vi "Measure_DUT_Capacitance.vi"(8 "error in":errorcluster, 9 "SoakTime":u16, 10 "AutoSoakFlag":u16) -> (0 "error out":errorcluster, 1 "data":string, 2 "Capacitance Data (in pF)":dbl format="%#.8g", 3 "Measure$":string)   [LabVIEW 2020]
uses:
  <vilib>/express/express arith-compare/Formula/XNode/ExpressFormulaBlockNode.xnode
panel:
  out "Total Time":i32
  out "Count":i32
  out "Qual 2 Data":dbl
  out "Qual Data":dbl
  out "Max Count":u32
  in  "DeltaCap!":dbl
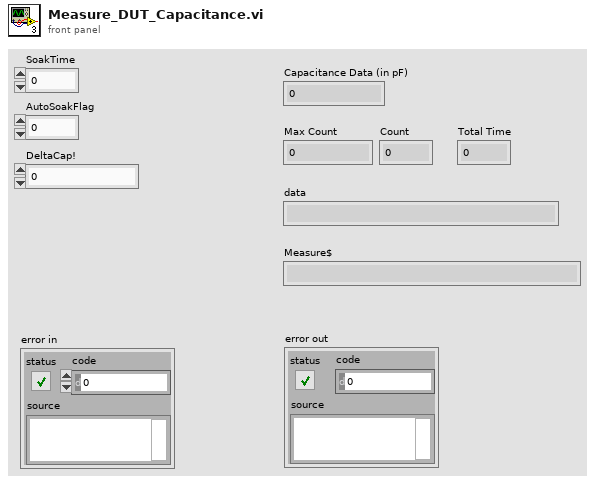
[diagram p1: front panel]
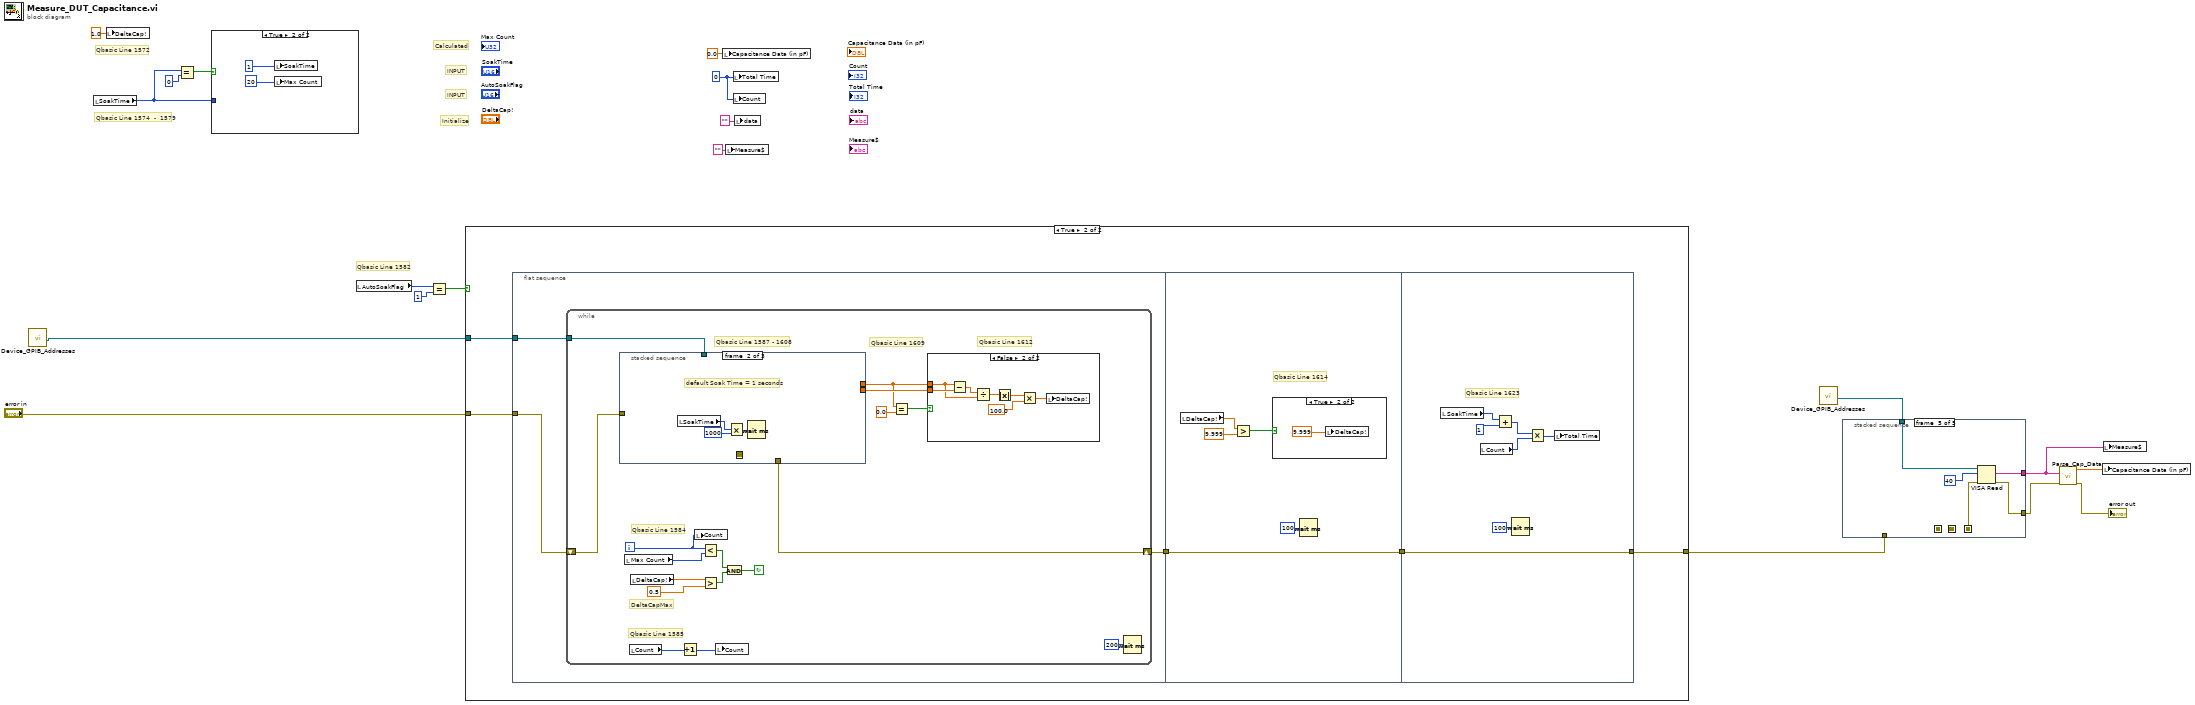
[diagram p0: block diagram]
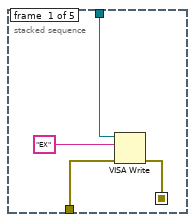
[diagram p2: hidden frame]
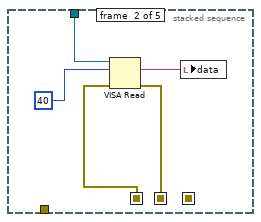
[diagram p3: hidden frame]
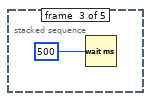
[diagram p4: hidden frame]
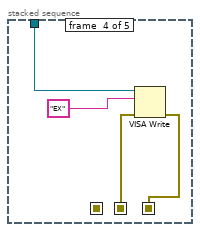
[diagram p5: hidden frame]
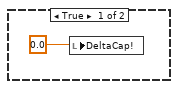
[diagram p7: hidden frame]
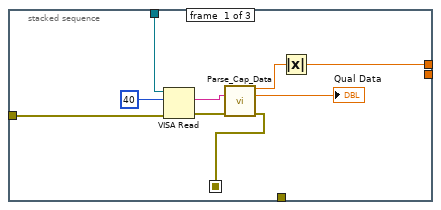
[diagram p8: hidden frame]
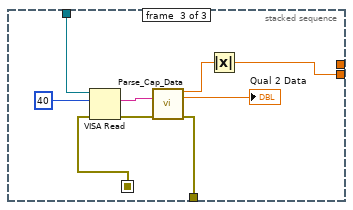
[diagram p9: hidden frame]
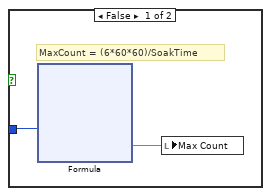
[diagram p11: hidden frame]
diagram:
  w4 = 0 ("Total Time")
  # "Initialize"
  # "Qbasic Line 1582"
  # "Calculated"
  # "Qbasic Line 1574  -  1579"
  # "INPUT"
  # "INPUT"
  # "Qbasic Line 1572"
  n1 = call "Device_GPIB_Addresses.vi"() -> ("HP 4275A Address"=w13:refnum<visa-resource-name>)  [unwired: 9 in, 2 out]
  n2 = local read "SoakTime"() -> (w8:u16)
  n3 = local write "DeltaCap!"(1.0 ("DeltaCap!")) -> ()
  n4 = Equal?(x=w8, y=0) -> (x = y?=w19:bool)
  n5 = case shown="True" w19 {
    tunnel: w8 -> [w21 _]
    frame False {
      # "MaxCount = (6*60*60)/SoakTime"
      n6 = xnode "Formula"("X1"=w21) -> ("Result"=w20:dbl)  [unwired: 1 in, 1 out]
      n7 = local write "Max Count"(w20) -> ()
    }
    frame True {
      n8 = local write "SoakTime"(1) -> ()
      n9 = local write "Max Count"(20) -> ()
    }
  }
  n10 = local read "AutoSoakFlag"() -> (w9:u16)
  n11 = Equal?(x=w9, y=u16 1) -> (x = y?=w16:bool)
  n12 = case shown="True" w16 {
    tunnel: "error in" -> [w32 w37]
    tunnel: [w32 w36] -> w15
    tunnel: w13 -> [_ w35]
    frame False {
    }
    frame True {
      n13 = flat-sequence {
        tunnel: w37 -> [w40]
        tunnel: w35 -> [w38]
        tunnel: [w39] -> w34
        tunnel: w34 -> [w91]
        tunnel: [w91] -> w33
        tunnel: [w99] -> w36
        tunnel: w33 -> [w99]
        frame #0 {
          n14 = while {
            tunnel: w38 -> [w46]
            shift-right: [w54] -> w39
            shift-left: w40 -> [w55]
            i -> [w41]
            stop <- w56 continue-if-true
            # "Qbasic Line 1609"
            # "Qbasic Line 1587 - 1608"
            # "Qbasic Line 1612"
            # "Qbasic Line 1585"
            # "Qbasic Line 1584"
            # "DeltaCapMax"
            n15 = stacked-sequence {
              seq-local: [w72 _ _] -> [_ _ w79]
              tunnel: w55 -> [w68 _ _]
              tunnel: [_ _ w85] -> w54
              tunnel: [_ _ w83] -> w53
              tunnel: [w71 _ _] -> w52
              tunnel: w46 -> [w70 _ w82]
              frame #0 {
                n16 = VISA Read(VISA resource name=w70, byte count=40, error in (no error)=w68) -> (read buffer=w67:string, error out=w66:errorcluster)  [unwired: 2 out]
                n17 = call "Parse_Cap_Data.vi"("Measure$"=w67, "error in"=w66) -> ("Capacitance Data (in pF)"=w74:dbl, "Qual Data"=→"Qual Data":dbl, "error out"=w72:errorcluster)  [unwired: 8 in, 3 out]
                n18 = Absolute Value(x=w74) -> (abs(x)=w71:dbl)
              }
              frame #1 {
                # "default Soak Time = 1 seconds"
                n19 = local read "SoakTime"() -> (w77:u16)
                n20 = Multiply(x=w77, y=u16 1000) -> (x*y=w75:u16)
                n21 = Wait (ms)(milliseconds to wait=w75) -> ()  [unwired: 1 out]
              }
              frame #2 {
                n22 = VISA Read(VISA resource name=w82, byte count=40, error in (no error)=w79) -> (read buffer=w78:string, error out=w80:errorcluster)  [unwired: 2 out]
                n23 = call "Parse_Cap_Data.vi"("Measure$"=w78, "error in"=w80) -> ("Capacitance Data (in pF)"=w86:dbl, "Qual Data"=→"Qual 2 Data":dbl, "error out"=w85:errorcluster)  [unwired: 8 in, 3 out]
                n24 = Absolute Value(x=w86) -> (abs(x)=w83:dbl)
              }
            }
            n25 = local read "Max Count"() -> (w49:u32)
            n26 = local read "Count"() -> (w45:i32)
            n27 = local read "DeltaCap!"() -> (w42:dbl)
            n28 = Increment(x=w45) -> (x+1=w44:i32)
            n29 = local write "Count"(w41) -> ()
            n30 = Less?(x=w41, y=w49) -> (x < y?=w48:bool)
            n31 = Greater?(x=w42, y=0.5 ("DeltaCapMax")) -> (0:w57:bool)
            n32 = local write "Count"(w44) -> ()
            n33 = And(x=w48, y=w57) -> (x .and. y?=w56:bool)
            n34 = Equal?(x=w52, y=0.0) -> (x = y?=w50:bool)
            n35 = case shown="False" w50 {
              tunnel: w53 -> [_ w65]
              tunnel: w52 -> [_ w63]
              frame True {
                n36 = local write "DeltaCap!"(0.0) -> ()
              }
              frame False {
                n37 = Subtract(x=w63, y=w65) -> (x-y=w64:dbl)
                n38 = Divide(x=w64, y=w63) -> (x/y=w62:dbl)
                n39 = Absolute Value(x=w62) -> (abs(x)=w61:dbl)
                n40 = Multiply(x=w61, y=100.0) -> (x*y=w59:dbl)
                n41 = local write "DeltaCap!"(w59) -> ()
              }
            }
            n42 = Wait (ms)(milliseconds to wait=u32 200) -> ()  [unwired: 1 out]
          }
        }
        frame #1 {
          # "Qbasic Line 1614"
          n43 = local read "DeltaCap!"() -> (w89:dbl)
          n44 = Greater?(x=w89, y=9.999) -> (0:w90:bool)
          n45 = case shown="True" w90 {
            frame False {
            }
            frame True {
              n46 = local write "DeltaCap!"(9.999 ("DeltaCap!")) -> ()
            }
          }
          n47 = Wait (ms)(milliseconds to wait=u32 100) -> ()  [unwired: 1 out]
        }
        frame #2 {
          # "Qbasic Line 1623"
          n48 = local read "SoakTime"() -> (w98:u16)
          n49 = local read "Count"() -> (w96:i32)
          n50 = Add(x=w98, y=u16 1) -> (x+y=w97:u16)
          n51 = Wait (ms)(milliseconds to wait=u32 100) -> ()  [unwired: 1 out]
          n52 = Multiply(x=w97, y=w96) -> (x*y=w93:i32)
          n53 = local write "Total Time"(w93) -> ()
        }
      }
    }
  }
  n54 = local write "Capacitance Data (in pF)"(0.0 ("Capacitance Data (in pF)")) -> ()
  n55 = local write "Measure$"("" ("data")) -> ()
  n56 = local write "Total Time"(w4) -> ()
  n57 = local write "Count"(w4) -> ()
  n58 = local write "data"("" ("data")) -> ()
  n59 = call "Device_GPIB_Addresses.vi"() -> ("HP 4275A Address"=w12:refnum<visa-resource-name>)  [unwired: 9 in, 2 out]
  n60 = stacked-sequence {
    seq-local: [w100 _ _ _ _] -> [_ w106 _ _ _]
    seq-local: [_ w105 _ _ _] -> [_ _ _ w112 _]
    seq-local: [_ _ _ w113 _] -> [_ _ _ _ w116]
    tunnel: w15 -> [w101 _ _ _ _]
    tunnel: w12 -> [w103 w108 _ w110 w118]
    tunnel: [_ _ _ _ w115] -> w11
    tunnel: [_ _ _ _ w114] -> w1
    frame #0 {
      n61 = VISA Write(VISA resource name=w103, write buffer="EX" ("data"), error in (no error)=w101) -> (error out=w100:errorcluster)  [unwired: 2 out]
    }
    frame #1 {
      n62 = VISA Read(VISA resource name=w108, byte count=40, error in (no error)=w106) -> (read buffer=w104:string, error out=w105:errorcluster)  [unwired: 2 out]
      n63 = local write "data"(w104) -> ()
    }
    frame #2 {
      n64 = Wait (ms)(milliseconds to wait=u32 500) -> ()  [unwired: 1 out]
    }
    frame #3 {
      n65 = VISA Write(VISA resource name=w110, write buffer="EX" ("data"), error in (no error)=w112) -> (error out=w113:errorcluster)  [unwired: 2 out]
    }
    frame #4 {
      n66 = VISA Read(VISA resource name=w118, byte count=40, error in (no error)=w116) -> (read buffer=w114:string, error out=w115:errorcluster)  [unwired: 2 out]
    }
  }
  n67 = call "Parse_Cap_Data.vi"("Measure$"=w1, "error in"=w11) -> ("Capacitance Data (in pF)"=w7:dbl, "error out"=→"error out":errorcluster)  [unwired: 8 in, 4 out]
  n68 = local write "Capacitance Data (in pF)"(w7) -> ()
  n69 = local write "Measure$"(w1) -> ()
